vi "2.2.vi"() -> ()   [LabVIEW 2017]
panel:
  out "Waveform Chart":dbl(graph)
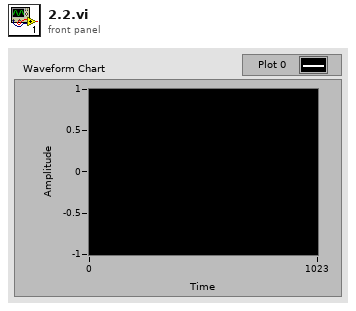
[diagram p1: front panel]
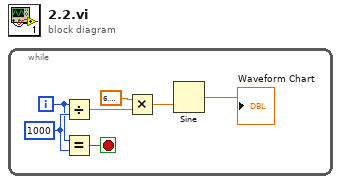
[diagram p0: block diagram]
diagram:
  n1 = while {
    i -> [w4]
    stop <- w7 stop-if-true
    w5 = 1000
    n2 = Divide(x=w4, y=w5) -> (x/y=w3:dbl)
    n3 = Equal?(x=w4, y=w5) -> (x = y?=w7:bool)
    n4 = Multiply(x=6.283185307179586, y=w3) -> (x*y=w2:dbl)
    n5 = Sine(x=w2) -> (sin(x)=→"Waveform Chart":dbl)
  }
